vi "Constructor.vi"(8 "error in (no error)":errorcluster, 11 "Aalborg GFC17 in":refnum<class "Aalborg GFC17.lvclass">) -> (0 "error out":errorcluster, 2 "Init":bool=TRUE, 3 "Aalborg GFC17 out":refnum<class "Aalborg GFC17.lvclass">)   [LabVIEW 2011, in "Aalborg GFC17.lvclass"]
uses:
  Aalborg GFC17.lvclass
  Aalborg GFC17.lvclass/Aalborg GFC17.ctl
  Mass Flow Controller/Valve Status.ctl
  <vilib>/DAQmx/create/channels.llb/DAQmx Create Channel (AO-Voltage-Basic).vi
  <vilib>/DAQmx/create/channels.llb/DAQmx Create Channel (AI-Voltage-Basic).vi
  Mass Flow Controller/Mass Flow Controller.lvclass
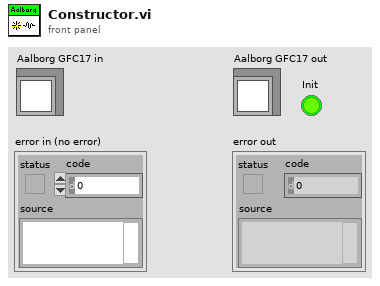
[diagram p1: front panel]
types:
  T1 = typedef "Mass Flow Controller.lvclass/Valve Status.ctl" = enum16{"Open", "Closed"}
  T2 = typedef "Aalborg GFC17.lvclass/Aalborg GFC17 Connections.ctl" = cluster{"flow rate setpoint channel":tag, "flow rate reading channel":tag, "valve channel":tag}
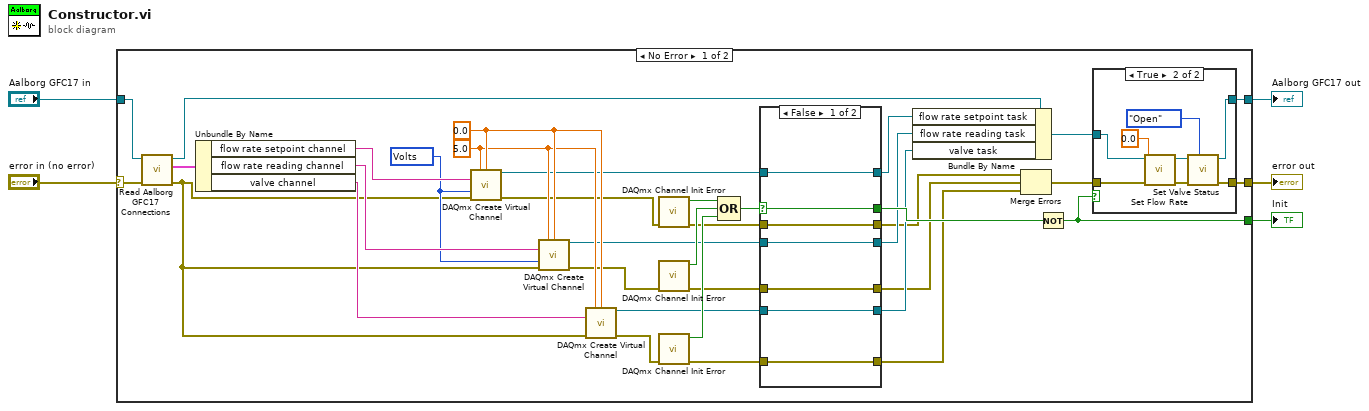
[diagram p0: block diagram]
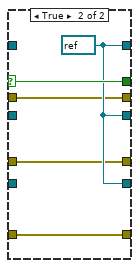
[diagram p3: hidden frame]
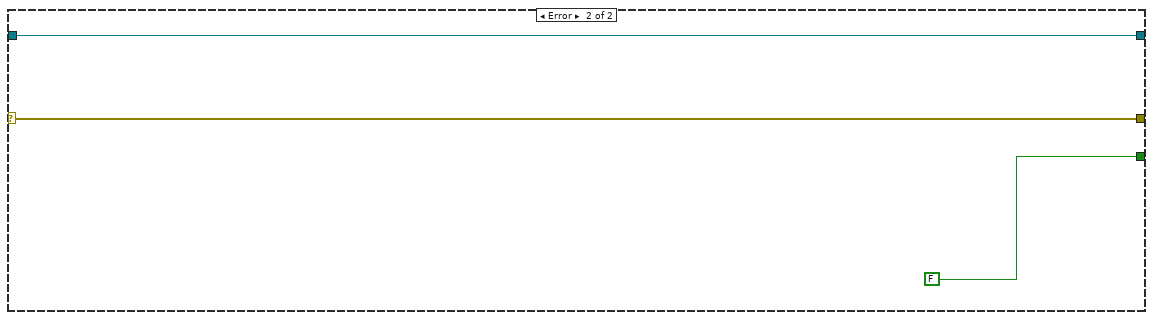
[diagram p4: hidden frame]
diagram:
  n1 = case shown="No Error" "error in (no error)" {
    selector: "error in (no error)" -> [w40 w66]
    tunnel: [w30 w66] -> w4
    tunnel: [w31 w65] -> w2
    tunnel: "Aalborg GFC17 in" -> [w39 w65]
    tunnel: [w6 FALSE ("status")] -> w1
    frame No Error {
      w33 = 10348 items=["Volts"=10348, "From Custom Scale"=10065] ("units")
      w29 = 0.0 ("minimum value")
      w28 = 5.0 ("maximum value")
      n2 = call-dynamic "Read Aalborg GFC17 Connections.vi"("error in (no error)"=w40, "Aalborg GFC17 in"=w39) -> ("error out"=w27:errorcluster, "Aalborg GFC17 Connections"=w37:T2, "Aalborg GFC17 out"=w38:refnum<class "Aalborg GFC17.lvclass">)  [unwired: 7 in]
      n3 = Unbundle By Name(w37) -> ("flow rate setpoint channel"=w36:tag, "flow rate reading channel"=w35:tag, "valve channel"=w34:tag)
      n4 = call-poly <vilib>:"DAQmx Create Virtual Channel.vi"("maximum value"=w28, "minimum value"=w29, "physical channels"=w36, "units"=w33, "error in"=w27) -> ("task out"=w15:refnum<k21>, "error out"=w25:errorcluster)  [unwired: 9 in]
      n5 = call-poly <vilib>:"DAQmx Create Virtual Channel.vi"("maximum value"=w28, "minimum value"=w29, "physical channels"=w35, "units"=w33, "error in"=w27) -> ("task out"=w14:refnum<k21>, "error out"=w26:errorcluster)  [unwired: 9 in]
      n6 = call-poly <vilib>:"DAQmx Create Virtual Channel.vi"("maximum value"=w28, "minimum value"=w29, "physical channels"=w34, "error in"=w27) -> ("task out"=w13:refnum<k21>, "error out"=w32:errorcluster)  [unwired: 10 in]
      n7 = call "DAQmx Channel Init Error.vi"("error in"=w25) -> ("error out"=w17:errorcluster, "channel init error?"=w24:bool)  [unwired: 9 in]
      n8 = call "DAQmx Channel Init Error.vi"("error in"=w26) -> ("error out"=w19:errorcluster, "channel init error?"=w23:bool)  [unwired: 9 in]
      n9 = call "DAQmx Channel Init Error.vi"("error in"=w32) -> ("error out"=w20:errorcluster, "channel init error?"=w22:bool)  [unwired: 9 in]
      n10 = Compound Arithmetic op=OR(w24, w23, w22) -> (w18:bool)
      n11 = case shown="False" w18 {
        selector: w18 -> [w55 w63]
        tunnel: w20 -> [w58 w59]
        tunnel: [w58 w59] -> w7
        tunnel: w19 -> [w57 w61]
        tunnel: [w57 w61] -> w8
        tunnel: w17 -> [w56 w60]
        tunnel: [w56 w60] -> w9
        tunnel: [w55 w63] -> w16
        tunnel: w15 -> [w54 _]
        tunnel: w14 -> [w53 _]
        tunnel: w13 -> [w52 _]
        tunnel: [w54 w62] -> w12
        tunnel: [w53 w62] -> w11
        tunnel: [w52 w62] -> w10
        frame False {
        }
        frame True {
          w62 = refnum<k21> refnum ("task out")
        }
      }
      n12 = Bundle By Name(cluster=w38, "flow rate setpoint task"=w12, "flow rate reading task"=w11, "valve task"=w10) -> (w41:refnum<class "Aalborg GFC17.lvclass">)
      n13 = Merge Errors(w9, w8, w7) -> (w21:errorcluster)
      n14 = Not(x=w16) -> (.not. x?=w6:bool)
      n15 = case shown="True" w6 {
        tunnel: w41 -> [w43 w51]
        tunnel: [w43 w46] -> w31
        tunnel: [w42 w45] -> w30
        tunnel: w21 -> [w42 w44]
        frame False {
        }
        frame True {
          n16 = call-dynamic "Set Flow Rate.vi"("error in (no error)"=w44, "Flow Rate"=0.0, "Aalborg GFC17 in"=w51) -> ("error out"=w50:errorcluster, "Aalborg GFC17 out"=w49:refnum<class "Aalborg GFC17.lvclass">)  [unwired: 7 in]
          n17 = call-dynamic "Set Valve Status.vi"("Valve Status"=Valve_Status."Open", "error in (no error)"=w50, "Aalborg GFC17 in"=w49) -> ("error out"=w45:errorcluster, "Aalborg GFC17 out"=w46:refnum<class "Aalborg GFC17.lvclass">)  [unwired: 7 in]
        }
      }
    }
    frame Error {
    }
  }
  "error out" <- w4
  "Aalborg GFC17 out" <- w2
  "Init" <- w1
